vi "Operations Monitor.vi"() -> ()   [LabVIEW 2016, in "Top Level.lvlib"]
doc: "This VI is part of the Top Level library of VIs that are opened upon startup. Vacuum pressures are read via serial connections between the vacuum gauge controller and the nearest cRIO. At the cRIO, a Real-Time VI puts the pressures into shared variables which are displayed here. \n\nThe individual cRIOs are pinged to check network connections and cRIO resources are from shared variables. \n\nThe Omega CNi854 Controller/Monitor measures temperature of Cs Oven on ion source and is communicated with directly over TCP."
uses:
  Top Level.lvlib
  <vilib>/Utility/miscctls.llb/LVRowAndColumnTypeDef.ctl
panel:
  in  "Tab Control":T1(tab)
  out "LE Waist":string
  out "Tank Entrance":string
  out "Tank Exit":string
  out "Analyzer Image":string
  out "HE Waist/Analyzer Object":string
  out "Transmission":string
  out "R30 Switch Image":string
  out "R30 Detector":string
  out "R30 ESA":string
  in  "stop":bool
  out "date/time string":string
  out "Injector A Image":string
  out "Injector A Object":string
  out "Terminal Voltage":dbl format="%#_4g"
  out "R45 EXB":string
  out "R45 Switch Image":string
  out "R45 Waist":string
  out "SCA bellows":string
  out "SCA source":string
  in  "Ping Timeout (ms)":i32=100
  out "cRIO Status":i32(listbox)
  out "Oven Temperature":dbl(graph)
  out "Oven Temp (°C)":dbl
  in  "Omega VISA resource":refnum<visa-resource-name>="TCPIP0::192.168.1.173::2000::SOCKET"
  out "Omega Iteration":i32
  in  "byte count":u32=15
  in  "Wait (ms)":u32=500
  out "Read errors":i32
  out "Omega read buffer":string
  out "SV read error":errorcluster
  out "Terminal read error":errorcluster
  out "Ping error":errorcluster
  in  "Clear Ping Error":bool
  out "cRIO SV error":errorcluster
  in  "Clear SV Error":bool
  out "Omega T error":errorcluster
  # "VACUUM  PRESSURES"
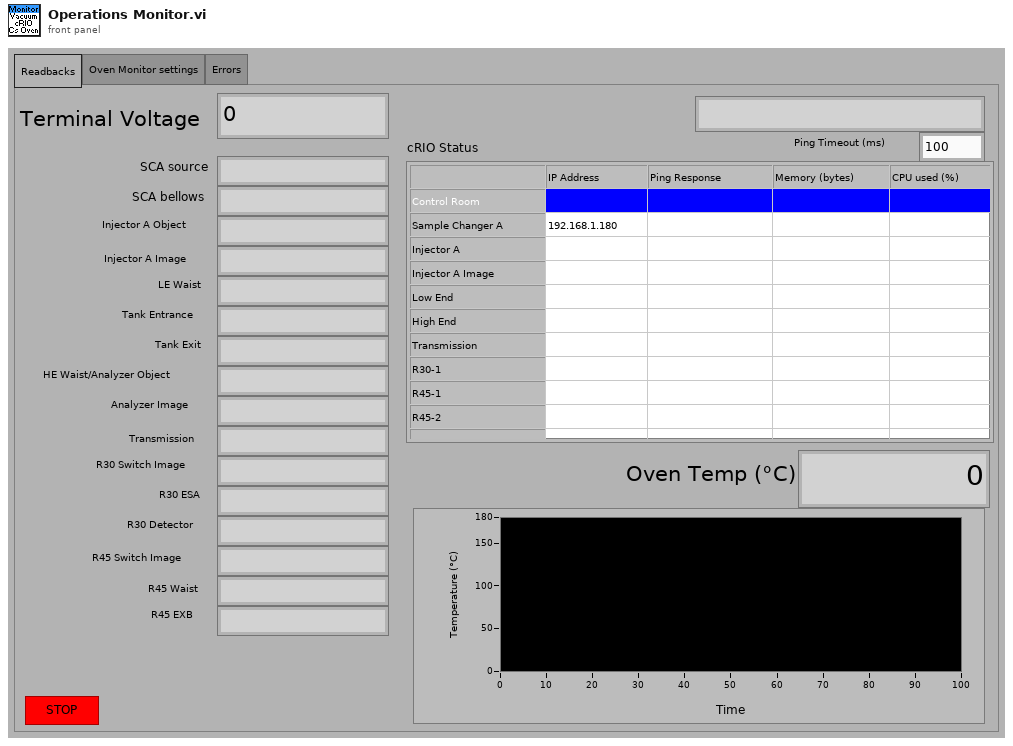
[diagram p1: front panel]
types:
  T1 = enum32{"Readbacks", "Oven Monitor settings", "Errors"}
  T2 = cluster{"Ion gauge 1":string, "Convectron  Gauge 1 ":string, "Ion Gauge 2":string, "Convectrom Gauge 2":string}
  T3 = typedef "LVRowAndColumnTypeDef.ctl" = cluster{"Row":i32, "Column":i32}
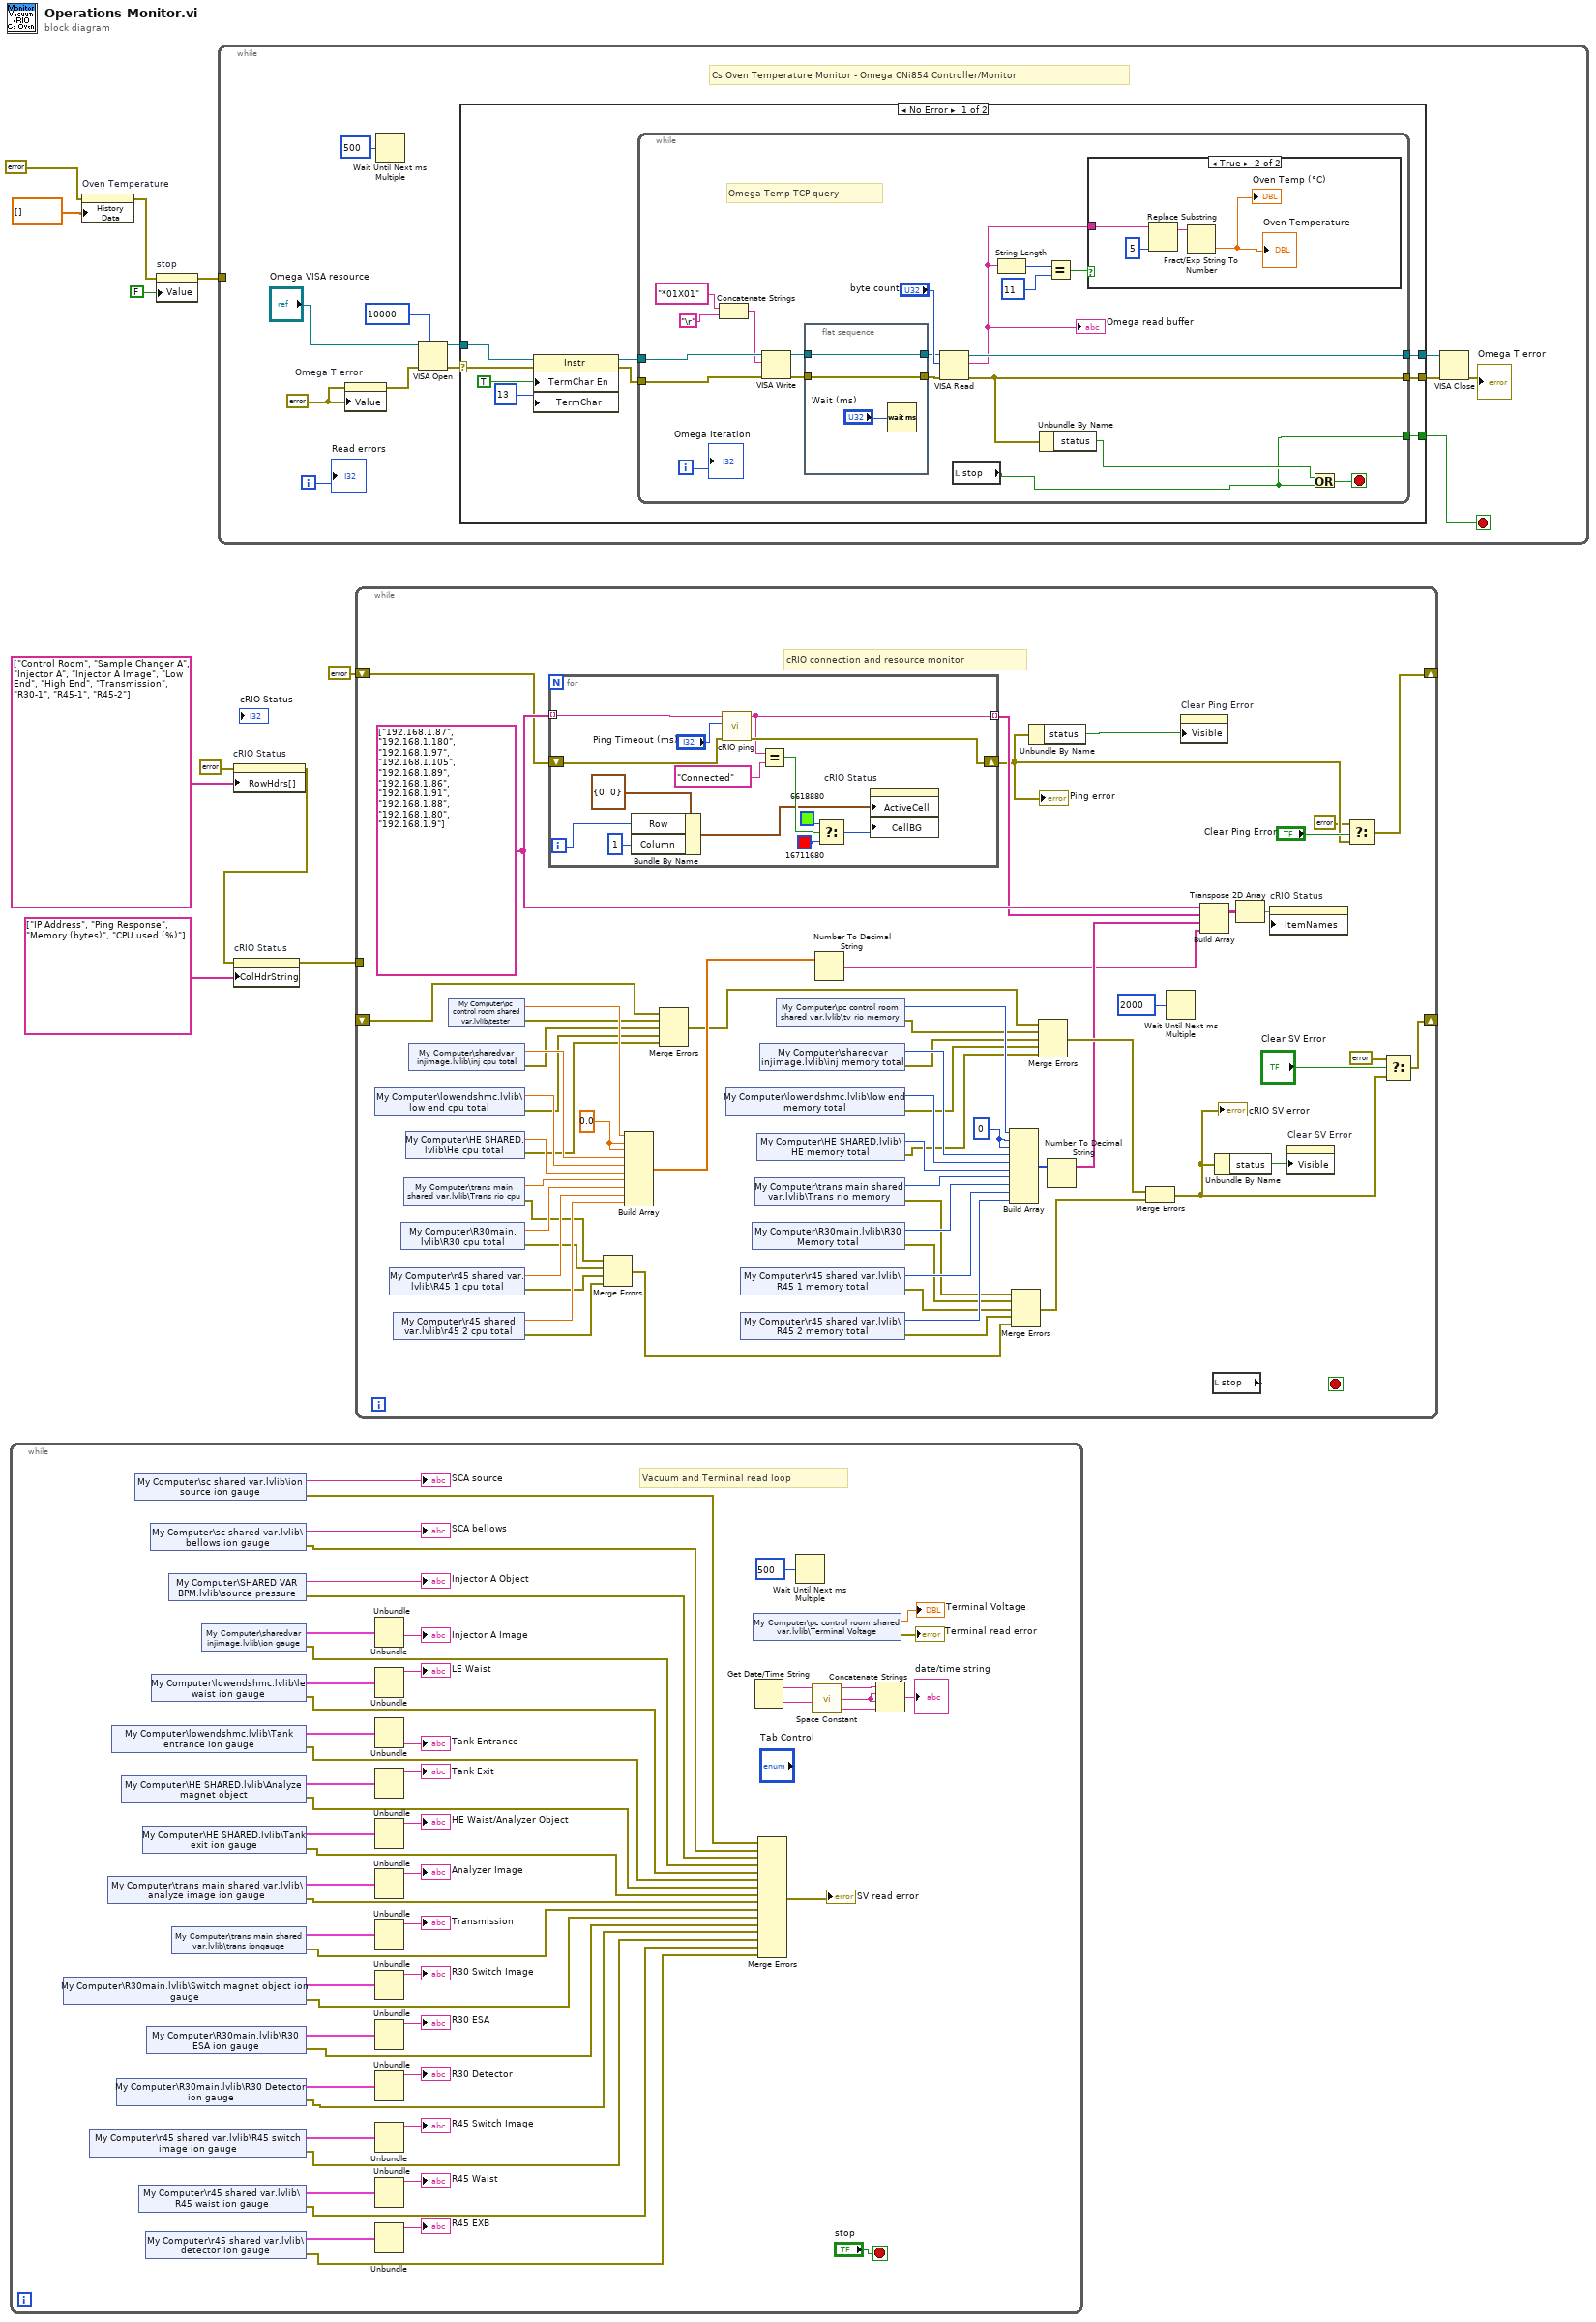
[diagram p0: block diagram]
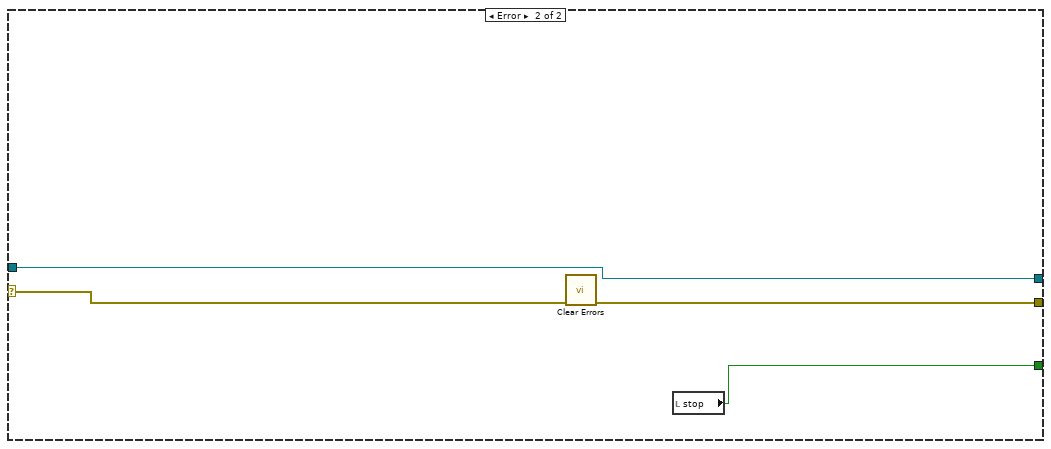
[diagram p3: hidden frame]
diagram:
  n1 = while {
    stop <- "stop" stop-if-true
    # "Vacuum and Terminal read loop"
    n2 = shared-variable "My Computer\\R30main.lvlib\\Switch magnet object ion gauge"() -> (w51:cluster{string, string, string, string}, error out=w18:errorcluster)  [unwired: 1 in]
    n3 = shared-variable "My Computer\\r45 shared var.lvlib\\R45 switch image ion gauge"() -> (w46:T2, error out=w15:errorcluster)  [unwired: 1 in]
    n4 = shared-variable "My Computer\\trans main shared var.lvlib\\analyze image ion gauge"() -> (w53:T2, error out=w20:errorcluster)  [unwired: 1 in]
    n5 = shared-variable "My Computer\\lowendshmc.lvlib\\Tank entrance ion gauge"() -> (w62:cluster{string, string, string, string}, error out=w23:errorcluster)  [unwired: 1 in]
    n6 = shared-variable "My Computer\\R30main.lvlib\\R30 Detector ion gauge"() -> (w50:cluster{string, string, string, string}, error out=w16:errorcluster)  [unwired: 1 in]
    n7 = shared-variable "My Computer\\HE SHARED.lvlib\\Analyze magnet object"() -> (w61:cluster{string, string, string, string}, error out=w22:errorcluster)  [unwired: 1 in]
    n8 = shared-variable "My Computer\\sc shared var.lvlib\\ion source ion gauge"() -> (→"SCA source":string, error out=w28:errorcluster)  [unwired: 1 in]
    n9 = shared-variable "My Computer\\r45 shared var.lvlib\\R45 waist ion gauge"() -> (w45:T2, error out=w14:errorcluster)  [unwired: 1 in]
    n10 = shared-variable "My Computer\\HE SHARED.lvlib\\Tank exit ion gauge"() -> (w60:cluster{string, string, string, string}, error out=w21:errorcluster)  [unwired: 1 in]
    n11 = shared-variable "My Computer\\r45 shared var.lvlib\\detector ion gauge"() -> (w47:T2, error out=w13:errorcluster)  [unwired: 1 in]
    n12 = shared-variable "My Computer\\R30main.lvlib\\R30 ESA ion gauge"() -> (w49:cluster{string, string, string, string}, error out=w17:errorcluster)  [unwired: 1 in]
    n13 = shared-variable "My Computer\\sc shared var.lvlib\\bellows ion gauge"() -> (→"SCA bellows":string, error out=w27:errorcluster)  [unwired: 1 in]
    n14 = shared-variable "My Computer\\lowendshmc.lvlib\\le waist ion gauge"() -> (w63:cluster{string, string, string, string}, error out=w24:errorcluster)  [unwired: 1 in]
    n15 = shared-variable "My Computer\\SHARED VAR BPM.lvlib\\source pressure"() -> (→"Injector A Object":string, error out=w26:errorcluster)  [unwired: 1 in]
    n16 = shared-variable "My Computer\\trans main shared var.lvlib\\trans iongauge"() -> (w52:T2, error out=w19:errorcluster)  [unwired: 1 in]
    n17 = shared-variable "My Computer\\sharedvar injimage.lvlib\\ion gauge"() -> (w59:cluster{string, string, string, string}, error out=w25:errorcluster)  [unwired: 1 in]
    n18 = Unbundle(w59) -> (→"Injector A Image":string)  [unwired: 3 out]
    n19 = Unbundle(w63) -> (→"LE Waist":string)  [unwired: 3 out]
    n20 = Unbundle(w62) -> (→"Tank Entrance":string)  [unwired: 3 out]
    n21 = Unbundle(w61) -> (→"Tank Exit":string)  [unwired: 3 out]
    n22 = Unbundle(w60) -> (→"HE Waist/Analyzer Object":string)  [unwired: 3 out]
    n23 = Unbundle(w53) -> ("Ion gauge 1"=→"Analyzer Image":string)  [unwired: 3 out]
    n24 = Unbundle(w52) -> ("Ion gauge 1"=→"Transmission":string)  [unwired: 3 out]
    n25 = Unbundle(w51) -> (→"R30 Switch Image":string)  [unwired: 3 out]
    n26 = Unbundle(w49) -> (→"R30 ESA":string)  [unwired: 3 out]
    n27 = Unbundle(w50) -> (→"R30 Detector":string)  [unwired: 3 out]
    n28 = Unbundle(w46) -> ("Ion gauge 1"=→"R45 Switch Image":string)  [unwired: 3 out]
    n29 = Unbundle(w45) -> ("Ion gauge 1"=→"R45 Waist":string)  [unwired: 3 out]
    n30 = Unbundle(w47) -> ("Ion gauge 1"=→"R45 EXB":string)  [unwired: 3 out]
    n31 = shared-variable "My Computer\\pc control room shared var.lvlib\\Terminal Voltage"() -> (→"Terminal Voltage":dbl, error out=→"Terminal read error":errorcluster)  [unwired: 1 in]
    n32 = Get Date/Time String() -> (date string=w57:string, time string=w54:string)  [unwired: 3 in]
    n33 = Merge Errors(w28, w27, w26, w25, w24, w23, w22, w21, w20, w19, w18, w17, w16, w15, w14, w13) -> (→"SV read error":errorcluster)
    n34 = Wait Until Next ms Multiple(millisecond multiple=u32 500) -> ()  [unwired: 1 out]
    n35 = call <vilib>:"Space Constant.vi"() -> ("String"=w55:string)
    n36 = Concatenate Strings(w57, w55, w55, w54) -> (→"date/time string":string)
  }
  n37 = property on="Oven Temperature" class="WFChart (strict)"(error in=errorcluster {"status"=FALSE, "code"=0, "source"=""} ("error in (no error)"), "History Data"=dbl[] []) -> (error out=w2:errorcluster)  [unwired: 1 in, 1 out]
  n38 = property on="stop" class="Bool (strict)"(error in=w2, "Value"=FALSE ("stop")) -> (error out=w1:errorcluster)  [unwired: 1 in, 1 out]
  n39 = while {
    tunnel: w1 -> [_]
    i -> [w69]
    stop <- w70 stop-if-true
    w72 = errorcluster {"status"=FALSE, "code"=0, "source"=""} ("error in (no error)")
    # "Cs Oven Temperature Monitor - Omega CNi854 Controller/Monitor"
    # "Omega Temperature Monitor Loop"
    n40 = property on="Omega T error" class="Clust (strict)"(error in=w72, "Value"=w72) -> (error out=w73:errorcluster)  [unwired: 1 in, 1 out]
    n41 = Wait Until Next ms Multiple(millisecond multiple=u32 500) -> ()  [unwired: 1 out]
    n42 = VISA Open(timeout (0)=u32 10000 ("VISA Open timeout (0)"), error in (no error)=w73, VISA resource name="Omega VISA resource") -> (VISA resource name=w77:refnum<visa-resource-name>, error out=w68:errorcluster)  [unwired: 2 in]
    n43 = case shown="No Error" w68 {
      selector: w68 -> [w79 w116]
      tunnel: w77 -> [w84 w117]
      tunnel: [w86 w117] -> w76
      tunnel: [w85 w115] -> w75
      tunnel: [w80 w114] -> w70
      frame No Error {
        n44 = property class="Instr"(reference=w84, error in=w79, "TermChar En"=TRUE ("Message Based Settings:Termination Character Enable"), "TermChar"=u8 13 ("Message Based Settings:Termination Character")) -> (reference out=w83:refnum<visa-resource-name>, error out=w78:errorcluster)
        n45 = while {
          tunnel: w83 -> [w102]
          tunnel: [w106] -> w86
          tunnel: w78 -> [w97]
          tunnel: [w105] -> w85
          tunnel: [w87] -> w80
          i -> [w103]
          stop <- w104 stop-if-true
          # "Omega Temp TCP query"
          n46 = Concatenate Strings("*01X01" ("data in"), "\r") -> (w99:string)
          n47 = VISA Write(VISA resource name=w102, write buffer=w99, error in (no error)=w97) -> (VISA resource name out=w90:refnum<visa-resource-name>, error out=w92:errorcluster)  [unwired: 1 out]
          n48 = flat-sequence {
            tunnel: w92 -> [w109]
            tunnel: [w109] -> w91
            tunnel: w90 -> [w108]
            tunnel: [w108] -> w89
            frame #0 {
              n49 = Wait (ms)(milliseconds to wait="Wait (ms)") -> ()  [unwired: 1 out]
            }
          }
          n50 = VISA Read(VISA resource name=w89, byte count="byte count", error in (no error)=w91) -> (VISA resource name out=w106:refnum<visa-resource-name>, read buffer=w93:string, error out=w105:errorcluster)  [unwired: 1 out]
          "Omega read buffer" <- w93
          n51 = local read "stop"() -> (w87:bool)
          n52 = String Length(string=w93) -> (length=w96:i32)
          n53 = Unbundle By Name(w105) -> ("status"=w88:bool)
          n54 = Equal?(x=w96, y=11) -> (x = y?=w94:bool)
          n55 = case shown="True" w94 {
            tunnel: w93 -> [_ w110]
            frame False {
            }
            frame True {
              n56 = Replace Substring(2:5 ("length (len. of substring)"), 5:w110) -> (1:w111:string)  [unwired: 2 in, 1 out]
              n57 = Fract/Exp String To Number(string=w111) -> (number=→"Oven Temp (°C)" →"Oven Temperature":dbl)  [unwired: 3 in, 1 out]
            }
          }
          n58 = Or(x=w88, y=w87) -> (x .or. y?=w104:bool)
          "Omega Iteration" <- w103
        }
      }
      frame Error {
        n59 = call <vilib>:"Clear Errors.vi"("error in (no error)"=w116) -> ("error out"=w115:errorcluster)  [unwired: 5 in, 1 out]
        n60 = local read "stop"() -> (w114:bool)
      }
    }
    n61 = VISA Close(VISA resource name=w76, error in (no error)=w75) -> (error out=→"Omega T error":errorcluster)
    "Read errors" <- w69
  }
  n62 = property on="cRIO Status" class="MCListbox (strict)"(error in=errorcluster {"status"=FALSE, "code"=0, "source"=""} ("error out"), "RowHdrs[]"=string[] ["Control Room", "Sample Changer A", "Injector A", "Injector A Image", "Low End", "High End", "Transmission", "R30-1", "R45-1", "R45-2"]) -> (error out=w6:errorcluster)  [unwired: 1 in, 1 out]
  n63 = property on="cRIO Status" class="MCListbox (strict)"(error in=w6, "ColHdrString"=string[] ["IP Address", "Ping Response", "Memory (bytes)", "CPU used (%)"]) -> (error out=w9:errorcluster)  [unwired: 1 in, 1 out]
  n64 = while {
    shift-right: [w122] -> _
    shift-left: _ -> [w147]
    shift-right: [w129] -> _
    shift-left: errorcluster {"status"=FALSE, "code"=0, "source"=""} ("Ping error out") -> [w154]
    tunnel: w9 -> [_]
    stop <- w120 stop-if-true
    w156 = string[] ["192.168.1.87", "192.168.1.180", "192.168.1.97", "192.168.1.105", "192.168.1.89", "192.168.1.86", "192.168.1.91", "192.168.1.88", "192.168.1.80", "192.168.1.9"]
    w157 = u32 0 ("element")
    w158 = 0.0 ("element")
    # "cRIO connection and resource monitor"
    n65 = shared-variable "My Computer\\lowendshmc.lvlib\\low end cpu total"() -> (w174:dbl, error out=w149:errorcluster)  [unwired: 1 in]
    n66 = shared-variable "My Computer\\r45 shared var.lvlib\\R45 1 cpu total"() -> (w170:dbl, error out=w146:errorcluster)  [unwired: 1 in]
    n67 = shared-variable "My Computer\\r45 shared var.lvlib\\r45 2 cpu total"() -> (w169:dbl, error out=w143:errorcluster)  [unwired: 1 in]
    n68 = shared-variable "My Computer\\R30main.lvlib\\R30 cpu total"() -> (w171:dbl, error out=w145:errorcluster)  [unwired: 1 in]
    n69 = shared-variable "My Computer\\trans main shared var.lvlib\\Trans rio cpu"() -> (w172:dbl, error out=w144:errorcluster)  [unwired: 1 in]
    n70 = shared-variable "My Computer\\HE SHARED.lvlib\\He cpu total"() -> (w173:dbl, error out=w148:errorcluster)  [unwired: 1 in]
    n71 = shared-variable "My Computer\\sharedvar injimage.lvlib\\inj cpu total"() -> (w175:dbl, error out=w150:errorcluster)  [unwired: 1 in]
    n72 = shared-variable "My Computer\\pc control room shared var.lvlib\\tester"() -> (w176:dbl, error out=w151:errorcluster)  [unwired: 1 in]
    n73 = for {
      tunnel: w156 -> [w190] mode=indexing
      tunnel: [w187] -> w155 mode=indexing
      shift-right: [w188] -> w127
      shift-left: w154 -> [w189]
      i -> [w180]
      n74 = Bundle By Name(cluster=T3 {"Row"=0, "Column"=0} ("Active Cell:Active Cell"), "Row"=w180, "Column"=1) -> (w179:T3)
      n75 = call "cRIO ping.vi"("Error in"=w189, "Ping Timeout (ms)"="Ping Timeout (ms)", "IP Address"=w190) -> ("Ping error out"=w188:errorcluster, "Ping Response"=w187:string)  [unwired: 7 in]
      n76 = Equal?(x=w187, y="Connected" ("t")) -> (x = y?=w184:bool)
      n77 = Select(t=u32 6618880, s=w184, f=u32 16711680) -> (s? t:f=w185:u32)
      n78 = property on="cRIO Status" class="MCListbox (strict)"("ActiveCell"=w179, "CellBG"=w185) -> ()  [unwired: 2 in, 2 out]
    }
    "Ping error" <- w127
    n79 = Merge Errors(w144, w145, w146, w143) -> (w132:errorcluster)
    n80 = Build Array(w176, w158, w158, w175, w174, w173, w172, w171, w170, w169) -> (w159:dbl[])
    n81 = Merge Errors(w147, w151, w150, w149, w148) -> (w142:errorcluster)
    n82 = shared-variable "My Computer\\lowendshmc.lvlib\\low end memory total"() -> (w162:u32, error out=w139:errorcluster)  [unwired: 1 in]
    n83 = shared-variable "My Computer\\r45 shared var.lvlib\\R45 1 memory total"() -> (w166:u32, error out=w136:errorcluster)  [unwired: 1 in]
    n84 = shared-variable "My Computer\\r45 shared var.lvlib\\R45 2 memory total"() -> (w167:u32, error out=w137:errorcluster)  [unwired: 1 in]
    n85 = shared-variable "My Computer\\R30main.lvlib\\R30 Memory total"() -> (w165:u32, error out=w135:errorcluster)  [unwired: 1 in]
    n86 = shared-variable "My Computer\\trans main shared var.lvlib\\Trans rio memory"() -> (w164:u32, error out=w134:errorcluster)  [unwired: 1 in]
    n87 = shared-variable "My Computer\\HE SHARED.lvlib\\HE memory total"() -> (w161:u32, error out=w138:errorcluster)  [unwired: 1 in]
    n88 = shared-variable "My Computer\\sharedvar injimage.lvlib\\inj memory total"() -> (w163:u32, error out=w140:errorcluster)  [unwired: 1 in]
    n89 = shared-variable "My Computer\\pc control room shared var.lvlib\\tv rio memory"() -> (w168:u32, error out=w141:errorcluster)  [unwired: 1 in]
    n90 = Number To Decimal String(number=w159) -> (decimal integer string=w118:string[])  [unwired: 1 in]
    n91 = Build Array(w168, w157, w157, w163, w162, w161, w164, w165, w166, w167) -> (w160:u32[])
    n92 = Merge Errors(w134, w135, w136, w137, w132) -> (w133:errorcluster)
    n93 = Unbundle By Name(w127) -> ("status"=w130:bool)
    n94 = Merge Errors(w142, w141, w140, w139, w138) -> (w131:errorcluster)
    n95 = Number To Decimal String(number=w160) -> (decimal integer string=w119:string[])  [unwired: 1 in]
    n96 = Merge Errors(w131, w133) -> (w121:errorcluster)
    "cRIO SV error" <- w121
    n97 = Wait Until Next ms Multiple(millisecond multiple=u32 2000) -> ()  [unwired: 1 out]
    n98 = property on="Clear Ping Error" class="Bool"("Visible"=w130) -> ()  [unwired: 2 in, 2 out]
    n99 = Build Array(w156, w155, w119, w118) -> (w153:string[][])
    n100 = local read "stop"() -> (w120:bool)
    n101 = Unbundle By Name(w121) -> ("status"=w125:bool)
    n102 = Transpose 2D Array(2D array=w153) -> (transposed array=w152:string[][])
    n103 = property on="cRIO Status" class="MCListbox (strict)"("ItemNames"=w152) -> ()  [unwired: 2 in, 2 out]
    n104 = property on="Clear SV Error" class="Bool"("Visible"=w125) -> ()  [unwired: 2 in, 2 out]
    n105 = Select(t=errorcluster {"status"=FALSE, "code"=0, "source"=""}, s="Clear Ping Error", f=w127) -> (s? t:f=w129:errorcluster)
    n106 = Select(t=errorcluster {"status"=FALSE, "code"=0, "source"=""}, s="Clear SV Error", f=w121) -> (s? t:f=w122:errorcluster)
  }
